vi "handle_errors.vi"(8 "error in (no error)":errorcluster, 11 "Action?":T1(ring)) -> (0 "error out":errorcluster)   [LabVIEW 2013]
uses:
  <vilib>/Utility/error.llb/DialogType.ctl
  Experiment/Globals.vi
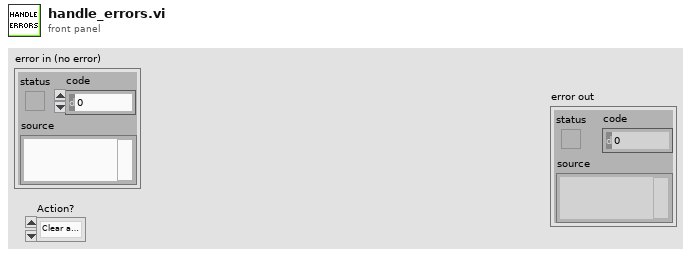
[diagram p1: front panel]
types:
  T1 = enum16{"Clear and Continue", "Clear and Restart", "Clear and Stop", "Halt"}
  T2 = typedef "DialogType.ctl" = u16
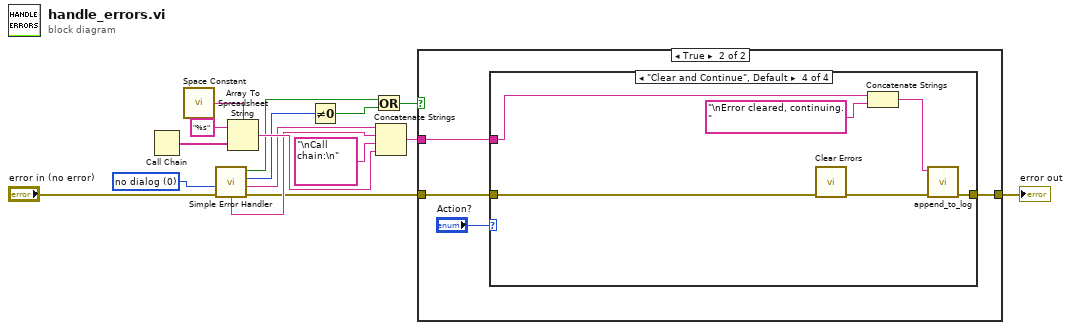
[diagram p0: block diagram]
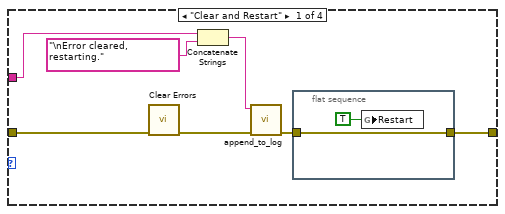
[diagram p3: hidden frame]
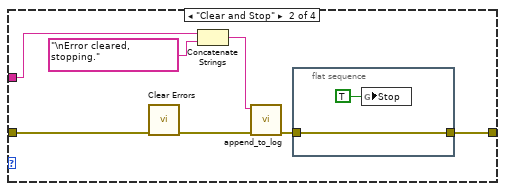
[diagram p4: hidden frame]
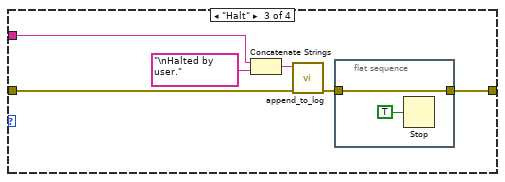
[diagram p5: hidden frame]
diagram:
  w7 = T2 0 items=["no dialog", "OK message", "continue or stop message", "OK message + warnings", "continue/stop + warnings"] ("type of dialog (OK msg:1)")
  n1 = Call Chain() -> (call chain=w12:string[])
  n2 = call <vilib>:"Space Constant.vi"() -> ("String"=w11:string)
  n3 = call <vilib>:"Simple Error Handler.vi"("type of dialog (OK msg:1)"=w7, "error in (no error)"="error in (no error)") -> ("error?"=w3:bool, "code out"=w2:i32, "source out"=w1:string, "error out"=w4:errorcluster, "message"=w5:string)  [unwired: 3 in]
  n4 = Array To Spreadsheet String(delimiter (Tab)=w11, array=w12, 3:"%s" ("format string")) -> (spreadsheet string=w10:string)
  n5 = Not Equal To 0?(x=w2) -> (x != 0?=w16:bool)
  n6 = Or(x=w3, y=w16) -> (x .or. y?=w15:bool)
  n7 = Concatenate Strings(w1, w5, "\nCall chain:\n" ("string"), w10) -> (w13:string)
  n8 = case shown="True" w15 {
    tunnel: w13 -> [_ w20]
    tunnel: [w17 w21] -> w14
    tunnel: w4 -> [w17 w19]
    frame False {
    }
    frame True {
      n9 = case shown="\"Clear and Continue\", Default" "Action?" {
        tunnel: w19 -> [w28 w32 w41 w50]
        tunnel: [w26 w37 w45 w48] -> w21
        tunnel: w20 -> [w24 w35 w44 w51]
        frame "Clear and Restart" {
          n10 = call <vilib>:"Clear Errors.vi"("error in (no error)"=w28) -> ("error out"=w27:errorcluster)  [unwired: 6 in]
          n11 = Concatenate Strings(w24, "\nError cleared, restarting." ("F button name (\"Cancel\")")) -> (w22:string)
          n12 = call "append_to_log.vi"("error in"=w27, "string"=w22) -> ("error out"=w25:errorcluster)  [unwired: 9 in]
          n13 = flat-sequence {
            tunnel: [w29] -> w26
            tunnel: w25 -> [w29]
            frame #0 {
              n14 = global write "Globals.vi" "Restart"(TRUE ("Restart")) -> ()
            }
          }
        }
        frame "Clear and Stop" {
          n15 = call <vilib>:"Clear Errors.vi"("error in (no error)"=w32) -> ("error out"=w31:errorcluster)  [unwired: 6 in]
          n16 = Concatenate Strings(w35, "\nError cleared, stopping." ("T button name (\"OK\")")) -> (w33:string)
          n17 = call "append_to_log.vi"("error in"=w31, "string"=w33) -> ("error out"=w36:errorcluster)  [unwired: 9 in]
          n18 = flat-sequence {
            tunnel: [w38] -> w37
            tunnel: w36 -> [w38]
            frame #0 {
              n19 = global write "Globals.vi" "Stop"(TRUE ("Stop")) -> ()
            }
          }
        }
        frame "Halt" {
          n20 = Concatenate Strings(w44, "\nHalted by user." ("T button name (\"OK\")")) -> (w42:string)
          n21 = call "append_to_log.vi"("error in"=w41, "string"=w42) -> ("error out"=w40:errorcluster)  [unwired: 9 in]
          n22 = flat-sequence {
            tunnel: [w46] -> w45
            tunnel: w40 -> [w46]
            frame #0 {
              n23 = Stop(stop? (T)=TRUE) -> ()
            }
          }
        }
        frame "Clear and Continue", Default {
          n24 = call <vilib>:"Clear Errors.vi"("error in (no error)"=w50) -> ("error out"=w49:errorcluster)  [unwired: 6 in]
          n25 = Concatenate Strings(w51, "\nError cleared, continuing." ("T button name (\"OK\")")) -> (w52:string)
          n26 = call "append_to_log.vi"("error in"=w49, "string"=w52) -> ("error out"=w48:errorcluster)  [unwired: 9 in]
        }
      }
    }
  }
  "error out" <- w14
